vi "Stop Core.vi"(10 "final error code":i32, 11 "IViewable in":refnum<class "IViewable.lvclass">) -> (3 "IViewable out":refnum<class "IViewable.lvclass">)   [LabVIEW 2015, in "IViewable.lvlib" / "IViewable.lvclass"]
doc: "(<B>Filename</B>: Actor Framework.lvlib:Actor.lvclass:Stop Core.vi)\n\nDefines what the actor does before it stops. Use the <B>final error code</B> input to determine whether the actor shut down in response to an error.\n\nBy default, this method does nothing. A descendant class may override it to define behavior, such as shutting down any processes the actor initiated in its override of the Actor Core method.\n\n<License>\nCopyright © 2017 Composed Systems, LLC | All rights reserved\nwww.composed.io\n\nAuthor: Ethan Stern <ethan.stern@composed.io>\n\nThis software is provided \"AS IS\" WITHOUT WARRANTIES, either express or implied, AND IS FOR EDUCATIONAL PURPOSES ONLY.\n</License>"
uses:
  IViewable.lvclass
  <vilib>/ActorFramework/Actor/Actor.lvclass/Actor.ctl
  IViewable.lvclass/IViewable.ctl
  <vilib>/ActorFramework/Message Enqueuer/Message Enqueuer.lvclass/Message Enqueuer.ctl
  IObserver/IObserver Messages/Unsubscribe Msg/Unsubscribe Msg.lvclass/Unsubscribe Msg.ctl
  <vilib>/ActorFramework/Actor/Read Self Enqueuer.vi
  <vilib>/ActorFramework/Message Enqueuer/Enqueue.vi
  <vilib>/ActorFramework/Message Enqueuer/Init from Existing Queue.vi
  <vilib>/ActorFramework/Message Priority Queue/Priority Enqueue.vi
  ActorEvents/IEventAggregator/IEventAggregator.lvclass
  <vilib>/ActorFramework/Message Enqueuer/Message Enqueuer.lvclass
  IObserver/IObserver Messages/Unsubscribe Msg/Unsubscribe Msg.lvclass
  <vilib>/ActorFramework/Actor/Actor.lvclass
  IObserver/IObserver/IObserver.lvclass
  ProtectedSubpanel/ProtectedSubpanel.lvclass
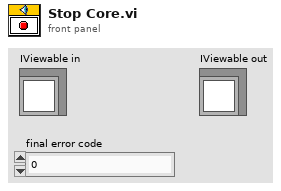
[diagram p1: front panel]
types:
  T1 = typedef "IViewable.lvlib/ProtectedSubpanel.lvclass/Protected Subpanel Reference.ctl" = refnum<data-value>
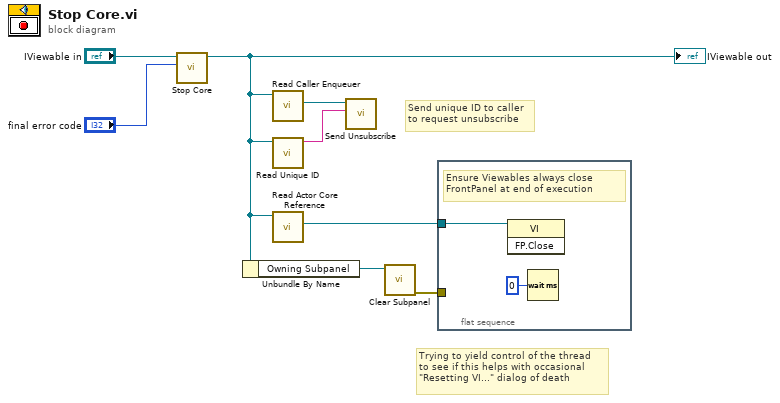
[diagram p0: block diagram]
diagram:
  # "Trying to yield control of the thread\nto see if this helps with occasional\n\"Resetting VI...\" dialog of death"
  # "Send unique ID to caller\nto request unsubscribe"
  n1 = call-parent "Stop Core.vi"("final error code"="final error code", "Actor in"="IViewable in") -> ("Actor out"=w3:refnum<class "IViewable.lvclass">)  [unwired: 9 in]
  "IViewable out" <- w3
  n2 = Unbundle By Name(w3) -> ("Owning Subpanel"=w2:T1)
  n3 = call <vilib>:"Read Caller Enqueuer.vi"("Actor"=w3) -> ("Caller Enqueuer"=w5:refnum<class "Message Enqueuer.lvclass">)  [unwired: 10 in]
  n4 = call "Read Unique ID.vi"("IObserver In"=w3) -> ("Unique ID"=w4:string)  [unwired: 10 in]
  n5 = call "Read Actor Core Reference.vi"("IViewable In"=w3) -> ("Actor Core Refnum"=w6:refnum<vi>)  [unwired: 9 in, 1 out]
  n6 = call "Send Unsubscribe.vi"("Unsubscriber ID"=w4, "Message Enqueuer"=w5) -> ()  [unwired: 8 in, 2 out]
  n7 = call "Clear Subpanel.vi"("Protected Subpanel"=w2) -> ("error out"=w1:errorcluster)  [unwired: 9 in, 1 out]
  n8 = flat-sequence {
    tunnel: w6 -> [w10]
    tunnel: w1 -> [_]
    frame #0 {
      # "Ensure Viewables always close\nFrontPanel at end of execution"
      n9 = invoke class="VI" method="FP.Close"(reference=w10) -> ()  [unwired: 2 in, 3 out]
      n10 = Wait (ms)(milliseconds to wait=u32 0) -> ()  [unwired: 1 out]
    }
  }
